vi "Server - Sensors.vi"() -> ()   [LabVIEW 2015]
panel:
  out "Error out 2":errorcluster
  out "data out":string
  in  "Number of Sensors":i32=20
  out "Messages Sent":dbl
  out "String length":i32
  in  "Wait [ms]":u32=10
  in  "Stop Sending":bool
  out "Message":string
  out "Error out":errorcluster
  in  "Timeout [ms]\n (wait forever: -1)":i32=-1
  in  "Port":u16=5555
  # "Server"
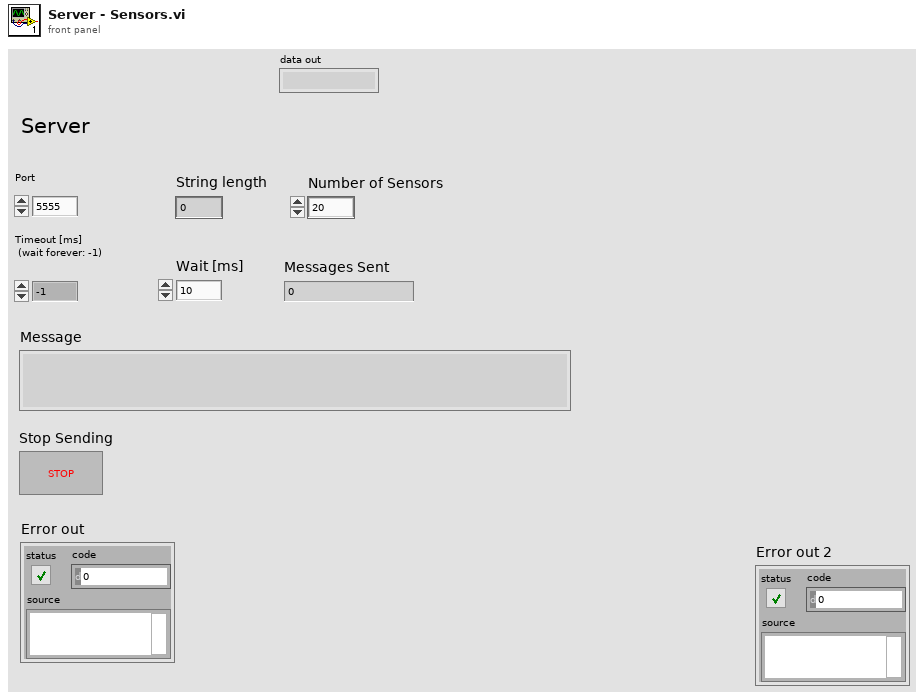
[diagram p1: front panel]
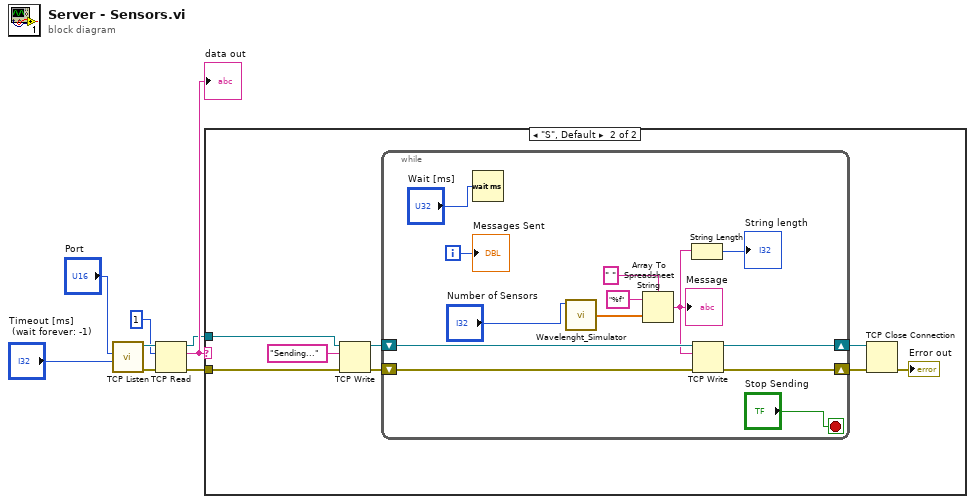
[diagram p0: block diagram]
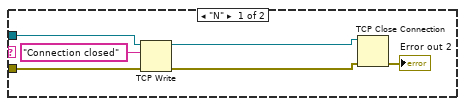
[diagram p2: hidden frame]
diagram:
  n1 = call <vilib>:"TCP Listen.vi"("timeout ms (wait forever: -1)"="Timeout [ms]\n (wait forever: -1)", "port"="Port") -> ("error out"=w5:errorcluster, "connection ID"=w6:refnum<k5>)  [unwired: 5 in, 3 out]
  n2 = TCP Read(connection ID=w6, bytes to read=1, error in (no error)=w5) -> (connection ID out=w2:refnum<k5>, data out=w3:string, error out=w1:errorcluster)  [unwired: 2 in]
  "data out" <- w3
  n3 = case shown="\"S\", Default" w3 {
    tunnel: w2 -> [w13 w19]
    tunnel: w1 -> [w12 w17]
    frame "N" {
      n4 = TCP Write(connection ID=w13, data in="Connection closed", error in (no error)=w12) -> (connection ID out=w9:refnum<k5>, error out=w10:errorcluster)  [unwired: 1 in, 1 out]
      n5 = TCP Close Connection(connection ID=w9, error in (no error)=w10) -> (error out=→"Error out 2":errorcluster)  [unwired: 1 in, 1 out]
    }
    frame "S", Default {
      n6 = TCP Write(connection ID=w19, data in="Sending...", error in (no error)=w17) -> (connection ID out=w18:refnum<k5>, error out=w16:errorcluster)  [unwired: 1 in, 1 out]
      n7 = while {
        shift-right: [w34] -> w21
        shift-left: w18 -> [w35]
        shift-right: [w32] -> w20
        shift-left: w16 -> [w33]
        i -> [w23]
        stop <- "Stop Sending" stop-if-true
        n8 = Wait (ms)(milliseconds to wait="Wait [ms]") -> ()  [unwired: 1 out]
        n9 = call "Wavelenght_Simulator.vi"("Number of Sensors"="Number of Sensors") -> ("Generated Wavelenghts"=w28:dbl[])  [unwired: 3 in]
        n10 = Array To Spreadsheet String(delimiter (Tab)=" ", array=w28, 3:"%f" ("format string")) -> (spreadsheet string=w25:string)
        "Message" <- w25
        n11 = String Length(string=w25) -> (length=→"String length":i32)
        n12 = TCP Write(connection ID=w35, data in=w25, error in (no error)=w33) -> (connection ID out=w34:refnum<k5>, error out=w32:errorcluster)  [unwired: 1 in, 1 out]
        "Messages Sent" <- w23
      }
      n13 = TCP Close Connection(connection ID=w21, error in (no error)=w20) -> (error out=→"Error out":errorcluster)  [unwired: 1 in, 1 out]
    }
  }
